vi "Make Vertical.vi"(8 "Matrix":T2 format="%.3f") -> (0 "Vertical Matrix":T2)   [LabVIEW 2013]
uses:
  <vilib>/Analysis/Matrix/Datatypes/RealMatrix.ctl
  <vilib>/Analysis/Matrix/NI_Matrix.lvlib
panel:
  out "XYZOAT 2":T1 {"Yaw" format="%.1f"; "Pitch" format="%.1f"; "Roll" format="%.1f"; "X" format="%.1f"}
  out "XYZOAT":T1
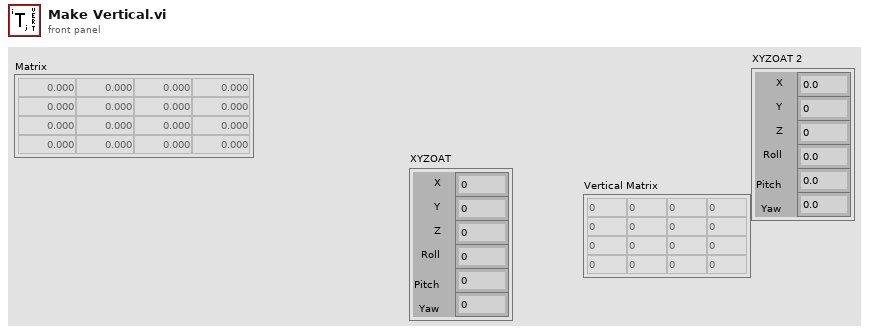
[diagram p1: front panel]
types:
  T1 = cluster{"X":dbl, "Y":dbl, "Z":dbl, "Roll":dbl, "Pitch":dbl, "Yaw":dbl}
  T2 = typedef "NI_Matrix.lvlib/RealMatrix.ctl" = dbl[][]
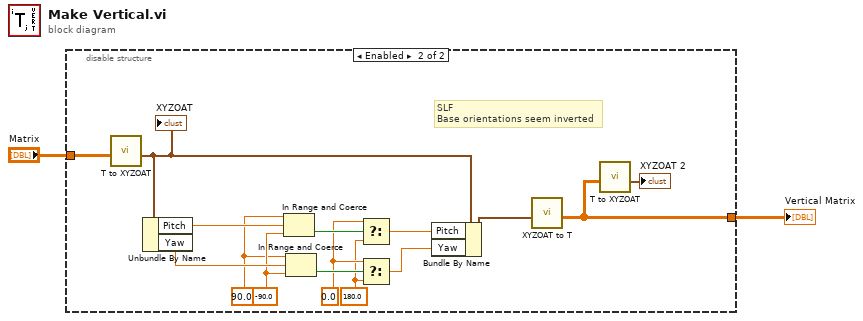
[diagram p0: block diagram]
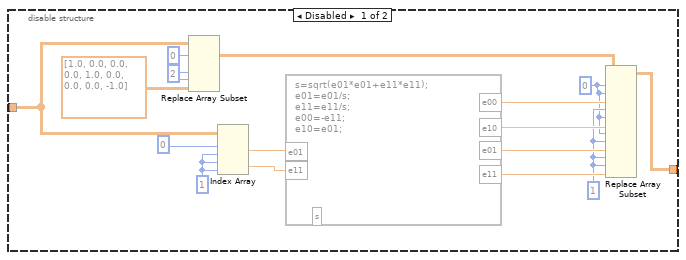
[diagram p2: hidden frame]
diagram:
  n1 = disable-structure shown="Enabled" {
    disable-tunnel: "Matrix" -> [w8 w32]
    disable-tunnel: [w3 w20] -> w1
    frame Disabled {
      w6 = 2 ("row N")
      w7 = 0 ("row 1")
      w10 = 1 ("disabled index (col)")
      w9 = 0 ("index (row)")
      w17 = 1 ("index (col)")
      n2 = Replace Array Subset(array=w8, new element=dbl[][] [[1.0, 0.0, 0.0], [0.0, 1.0, 0.0], [0.0, 0.0, -1.0]], index (dim 0)=w7, index (dim 1)=w6, index (dim 2)=w7, index (dim 3)=w6) -> (w4:T2)
      n3 = Index Array(array=w8, index (row) #1=0 ("row 1"), index (col) #1=w17, index (row) #2=w17, index (col) #2=w17) -> (element #1=w16:dbl, element #2=w15:dbl)
      n4 = formula code="s=sqrt(e01*e01+e11*e11);\ne01=e01/s;\ne11=e11/s;\ne00=-e11;\ne10=e01;"("e01"=w16, "e11"=w15) -> ("e01"=w11:dbl, "e11"=w12:dbl, "e00"=w14:dbl, "e10"=w13:dbl)  [unwired: 1 out]
      n5 = Replace Array Subset(array=w4, new element #1=w14, index (row) #1=w9, index (col) #1=w9, new element #2=w13, index (row) #2=w10, index (col) #2=w9, new element #3=w11, index (row) #3=w9, index (col) #3=w10, new element #4=w12, index (row) #4=w10, index (col) #4=w10) -> (w3:T2)
    }
    frame Enabled {
      w23 = 180.0 ("Pitch")
      w24 = 0.0 ("Pitch")
      w22 = -90.0 ("lower limit")
      w21 = 90.0 ("upper limit")
      # "SLF\nBase orientations seem inverted"
      n6 = call "T to XYZOAT.vi"("T"=w32) -> ("XYZOAT"=w30:T1)  [unwired: 10 in]
      "XYZOAT" <- w30
      n7 = Unbundle By Name(w30) -> ("Pitch"=w26:dbl, "Yaw"=w31:dbl)
      n8 = In Range and Coerce(upper limit=w21, x=w26, lower limit=w22) -> (In Range?=w27:bool)  [unwired: 1 out]
      n9 = In Range and Coerce(upper limit=w21, x=w31, lower limit=w22) -> (In Range?=w29:bool)  [unwired: 1 out]
      n10 = Select(t=w24, s=w27, f=w23) -> (s? t:f=w25:dbl)
      n11 = Select(t=w24, s=w29, f=w23) -> (s? t:f=w28:dbl)
      n12 = Bundle By Name(cluster=w30, "Pitch"=w25, "Yaw"=w28) -> (w33:T1)
      n13 = call "XYZOAT to T.vi"("XYZOAT"=w33) -> ("T"=w20:T2)  [unwired: 10 in]
      n14 = call "T to XYZOAT.vi"("T"=w20) -> ("XYZOAT"=→"XYZOAT 2":T1)  [unwired: 10 in]
    }
  }
  "Vertical Matrix" <- w1
